vi "DataLogger.ProcCases.vi"(0 "i ref in":refnum<vi>, 1 "selector":string, 2 "Data":T1, 3 "call cluster":T2={"Object"="", "Selector"="", "CallType"=enum."synchronous", "Async Object"="", "Async Selector"="", "Data Descriptor"="", "Data"=[], "Error #"=0, "Expire"=0}, 5 "error in (no error)":errorcluster) -> (14 "i ref out":refnum<vi>, 17 "answer cluster":T2={"Object"="", "Selector"="", "CallType"=enum."synchronous", "Async Object"="", "Async Selector"="", "Data Descriptor"="", "Data"=[], "Error #"=0, "Expire"=0}, 19 "error out":errorcluster)   [LabVIEW 2014, in "DataLogger.lvlib"]
doc: "This method is called by a process from within the default case in the event loop. The methods of a class that are linked to events will be called from THIS method. Add your code here."
uses:
  DataLogger.lvlib
  CS_Core/CSSystem/CoreDefs/CoreDefs.call_type.ctl
  CS_Core/BaseProcess/BaseProcess.descriptor string definition.ctl
  CS_Core/CSSystem/CoreDefs/CoreDefs.rawDataType.ctl
  CS_Core/CSSystem/CoreLib/CoreLib.byte array 2 double.vi
  CS_Core/CSSystem/CoreLib/CoreLib.double 2 byte array.vi
  CS_Core/CSSystem/CoreLib/CoreLib.string 2 byte array.vi
  CS_Core/CSSystem/CoreLib/CoreLib.lvlib
  CS_Core/BaseProcess/BaseProcess.lvlib
  CS_Core/CSApplicationBaseClasses/DeviceBase/DeviceBase.lvlib
  CS_Core/CAEObj/CAEObj.lvlib
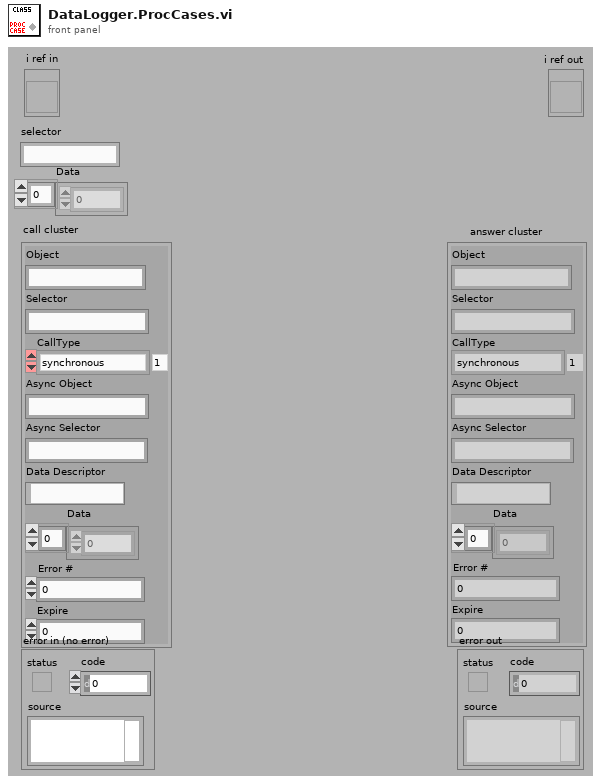
[diagram p1: front panel]
types:
  T1 = typedef "CoreDefs.rawDataType.ctl" = i8[]
  T2 = typedef "CoreDefs.call_type.ctl" = cluster{"Object":string, "Selector":string, "CallType":enum16{"simple", "synchronous", "asynchronous"}, "Async Object":string, "Async Selector":string, "Data Descriptor":T3, "Data":T1, "Error #":i32, "Expire":u32}
  T3 = typedef "BaseProcess.lvlib/BaseProcess.descriptor string definition.ctl" = string
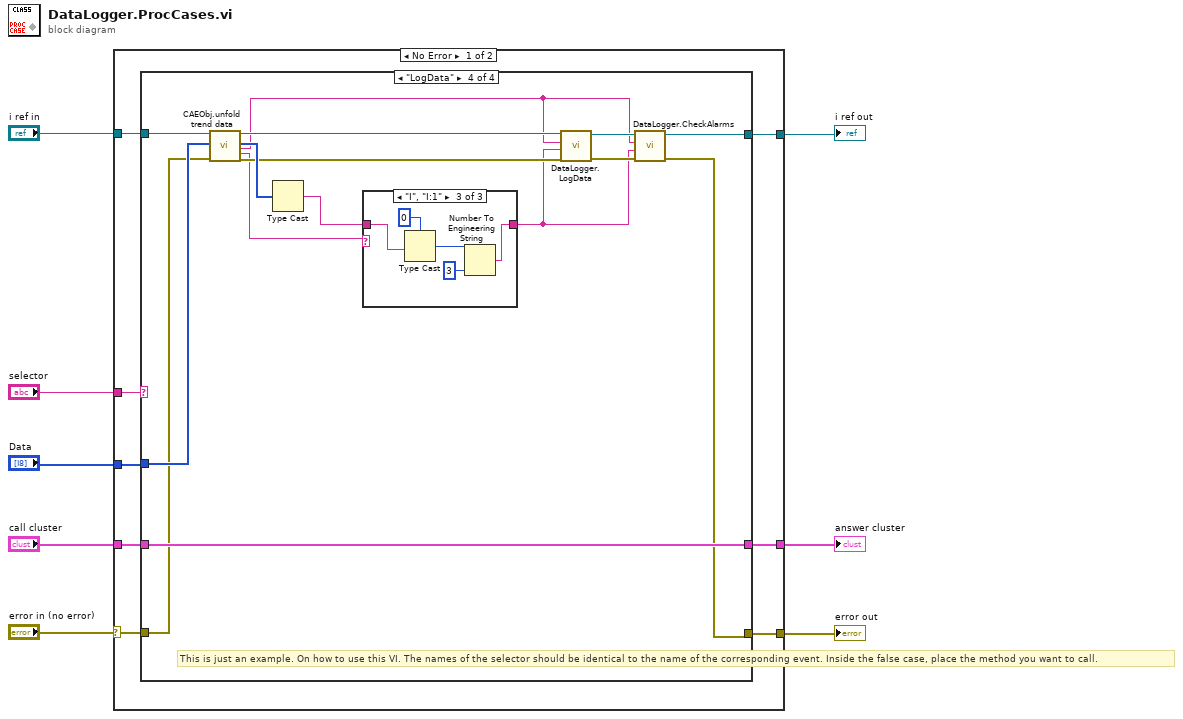
[diagram p0: block diagram]
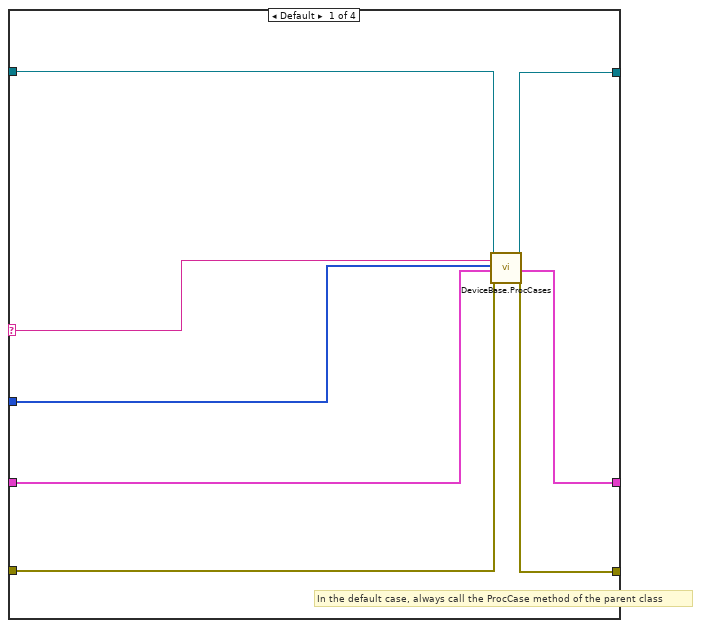
[diagram p2: hidden frame]
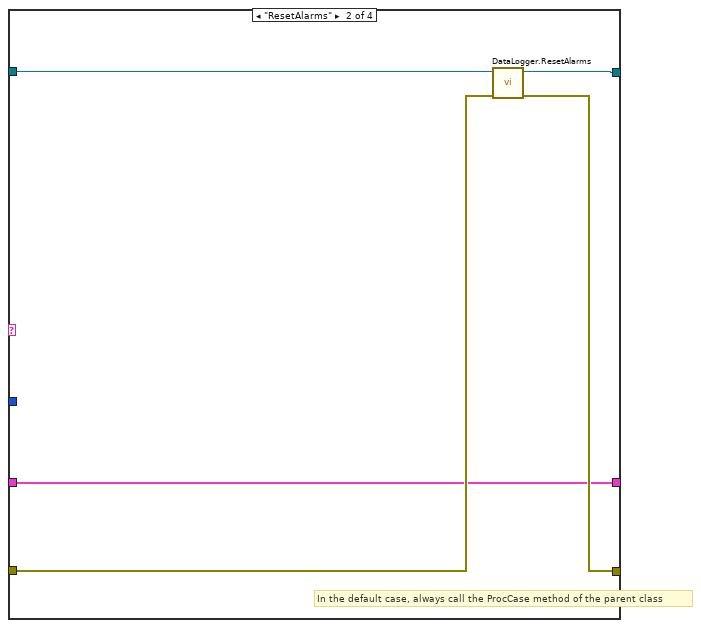
[diagram p3: hidden frame]
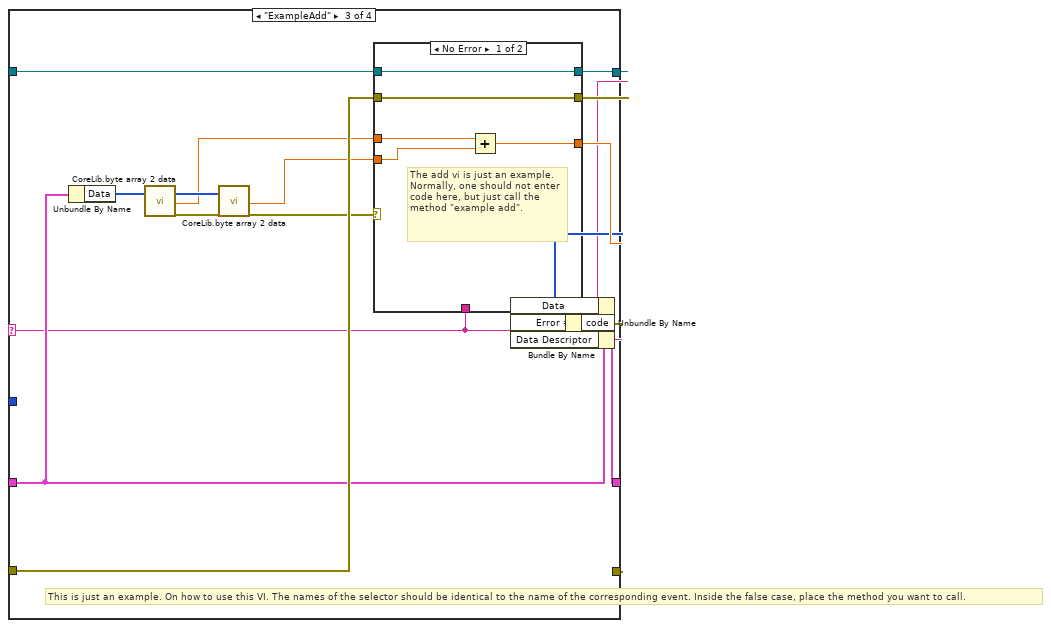
[diagram p4: hidden frame]
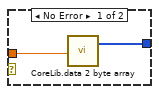
[diagram p5: hidden frame]
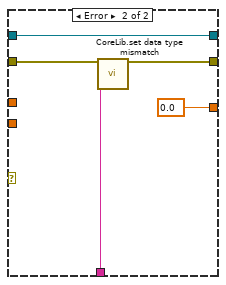
[diagram p6: hidden frame]
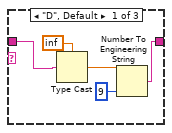
[diagram p7: hidden frame]
diagram:
  n1 = case shown="No Error" "error in (no error)" {
    selector: "error in (no error)" -> [w9 w90]
    tunnel: "selector" -> [w16 _]
    tunnel: [w15 w91] -> w7
    tunnel: "Data" -> [w14 _]
    tunnel: "call cluster" -> [w13 w91]
    tunnel: "i ref in" -> [w12 w92]
    tunnel: [w11 w92] -> w3
    tunnel: [w10 w90] -> w2
    frame No Error {
      n2 = case shown="\"LogData\"" w16 {
        selector: w16 -> [w19 _ w38 _]
        tunnel: w14 -> [w17 _ _ w78]
        tunnel: w12 -> [w18 w29 w48 w77]
        tunnel: [w24 w28 w37 w68] -> w11
        tunnel: w13 -> [w20 w25 w44 w76]
        tunnel: [w21 w25 w43 w76] -> w15
        tunnel: w9 -> [w23 w27 w47 w73]
        tunnel: [w22 w26 w39 w66] -> w10
        frame Default {
          # "In the default case, always call the ProcCase method of the parent class"
          n3 = call "DeviceBase.ProcCases.vi"("i ref in"=w18, "selector"=w19, "Data"=w17, "call cluster"=w20, "error in (no error)"=w23) -> ("i ref out"=w24:refnum<vi>, "answer cluster"=w21:T2, "error out"=w22:errorcluster)  [unwired: 12 in]
        }
        frame "ResetAlarms" {
          # "In the default case, always call the ProcCase method of the parent class"
          n4 = call "DataLogger.ResetAlarms.vi"("error in (no error)"=w27, "i ref in"=w29) -> ("error out"=w26:errorcluster, "i ref out"=w28:refnum<vi>)  [unwired: 8 in]
        }
        frame "ExampleAdd" {
          # "This is just an example. On how to use this VI. The names of the selector should be identical to the name of the corresponding event. Inside the false case, place the method you want to call."
          n5 = Unbundle By Name(w44) -> ("Data"=w35:T1)
          n6 = call-poly "CoreLib.byte array 2 data.vi"("byteArray"=w35) -> ("byteArray out"=w33:T1, "d64"=w31:dbl, "error out"=w34:errorcluster)  [unwired: 16 in]
          n7 = call-poly "CoreLib.byte array 2 data.vi"("byteArray"=w33, "error in (no error)"=w34) -> ("d64"=w30:dbl, "error out"=w32:errorcluster)  [unwired: 15 in, 1 out]
          n8 = case shown="No Error" w32 {
            tunnel: [w55 w63] -> w41
            tunnel: w48 -> [w55 w63]
            tunnel: w47 -> [w56 w62]
            tunnel: [w56 w61] -> w40
            tunnel: w30 -> [w58 _]
            tunnel: [w57 0.0] -> w46
            tunnel: w38 -> [_ w59]
            tunnel: w31 -> [w54 _]
            frame No Error {
              # "The add vi is just an example. Normally, one should not enter code here, but just call the method \"example add\"."
              n9 = Add(x=w54, y=w58) -> (x+y=w57:dbl)
            }
            frame Error {
              n10 = call "CoreLib.set data type mismatch.vi"("error in (no error)"=w62, "error source"=w59) -> ("error out"=w61:errorcluster)  [unwired: 17 in]
            }
          }
          n11 = call "BaseProcess.set event status.vi"("i ref in"=w41, "EventStatus"=w38, "error in (no error)"=w40) -> ("i ref out"=w37:refnum<vi>, "error out"=w39:errorcluster)  [unwired: 14 in, 1 out]
          n12 = Unbundle By Name(w39) -> ("code"=w45:i32)
          n13 = case shown="Error" w39 {
            selector: w39 -> [_ w53]
            tunnel: [w49 w52] -> w42
            tunnel: w46 -> [w50 _]
            frame No Error {
              n14 = call-poly "CoreLib.data 2 byte array.vi"("f64"=w50) -> ("byteArray out"=w49:T1)  [unwired: 18 in]
            }
            frame Error {
              n15 = Unbundle By Name(w53) -> ("source"=w51:string)
              n16 = call-poly "CoreLib.data 2 byte array.vi"("string"=w51) -> ("byteArray out"=w52:T1)  [unwired: 18 in]
            }
          }
          n17 = Bundle By Name(cluster=w44, "Data"=w42, "Error #"=w45, "Data Descriptor"="D:1") -> (w43:T2)
        }
        frame "LogData" {
          # "This is just an example. On how to use this VI. The names of the selector should be identical to the name of the corresponding event. Inside the false case, place the method you want to call."
          n18 = call "CAEObj.unfold trend data.vi"("i ref in"=w77, "raw trend data"=w78, "error in (no error)"=w73) -> ("i ref out"=w75:refnum<vi>, "data"=w74:i8[], "serviceName"=w65:string, "typeDescriptor"=w71:string, "error out"=w72:errorcluster)  [unwired: 8 in, 4 out]
          n19 = Type Cast(x=w74) -> (*(type *) &x=w70:string)  [unwired: 1 in]
          n20 = case shown="\"I\", \"I:1\"" w71 {
            tunnel: [w80 w84 w85] -> w64
            tunnel: w70 -> [w79 w84 w86]
            frame "D", Default {
              n21 = Type Cast(type=inf, x=w79) -> (*(type *) &x=w82:dbl)
              n22 = Number To Engineering String(2:i16 9 ("precision (6)"), 4:w82) -> (0:w80:string)  [unwired: 2 in]
            }
            frame "C" {
            }
            frame "I", "I:1" {
              n23 = Type Cast(type=0, x=w86) -> (*(type *) &x=w88:i32)
              n24 = Number To Engineering String(2:i16 3 ("precision (6)"), 4:w88) -> (0:w85:string)  [unwired: 2 in]
            }
          }
          n25 = call "DataLogger.LogData.vi"("error in (no error)"=w72, "Value"=w64, "DIM Service"=w65, "i ref in"=w75) -> ("error out"=w67:errorcluster, "i ref out"=w69:refnum<vi>)  [unwired: 6 in]
          n26 = call "DataLogger.CheckAlarms.vi"("error in (no error)"=w67, "Value"=w64, "DIM Service"=w65, "i ref in"=w69) -> ("error out"=w66:errorcluster, "i ref out"=w68:refnum<vi>)  [unwired: 6 in]
        }
      }
    }
    frame Error {
    }
  }
  "answer cluster" <- w7
  "i ref out" <- w3
  "error out" <- w2
